vi "DebugCam_GetSize.vi"(8 "error in (no error)":errorcluster) -> (0 "error out":errorcluster, 1 "h":i32=320, 2 "w":i32=480, 3 "status":i32)   [LabVIEW 2014, in "QwaveSys RPi Training Library.lvlib"]
uses:
  <vilib>/Q-Wave Systems/QwaveSys RPi Training Package (Demo)/Addons/QwaveSys RPi Training Library.lvlib
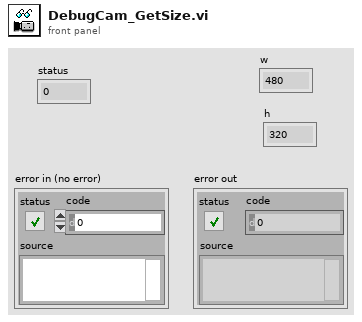
[diagram p1: front panel]
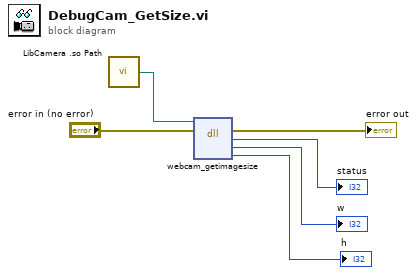
[diagram p0: block diagram]
diagram:
  n1 = call <vilib>:"LibCamera .so Path.vi"() -> ("LibCam .so Path"=w4:path)  [unwired: 5 in]
  n2 = dll-call lib="libcamera.so" fn="webcam_getimagesize"(path in=w4, error in="error in (no error)") -> (error out=→"error out":errorcluster, "return type"=→"status":i32, "w"=→"w":i32, "h"=→"h":i32)  [unwired: 3 in, 1 out]
